vi "Bus Wiring.vi"(6 "Variant in":variant, 7 "Shift Pressed?":bool, 8 "error in (no error)":errorcluster, 10 "QD Combo Box Ref":refnum<vi>, 11 "QD Launch VI Ref":refnum<vi>) -> (0 "error out":errorcluster, 4 "Variant out":variant)   [LabVIEW 2019]
doc: "Attempt to bus wires\n\nDefault Shortcut - [e]"
panel:
  in  "Undo Name":string="Reset to Origin"
  # "Do not change the connector pane of this VI.\n\nSee the block diagram for directions on how to use this template."
  # "Specify the name of the Undo transaction"
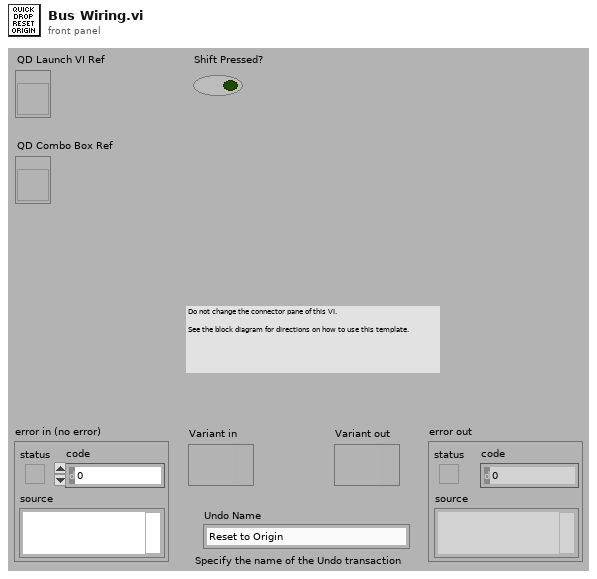
[diagram p1: front panel]
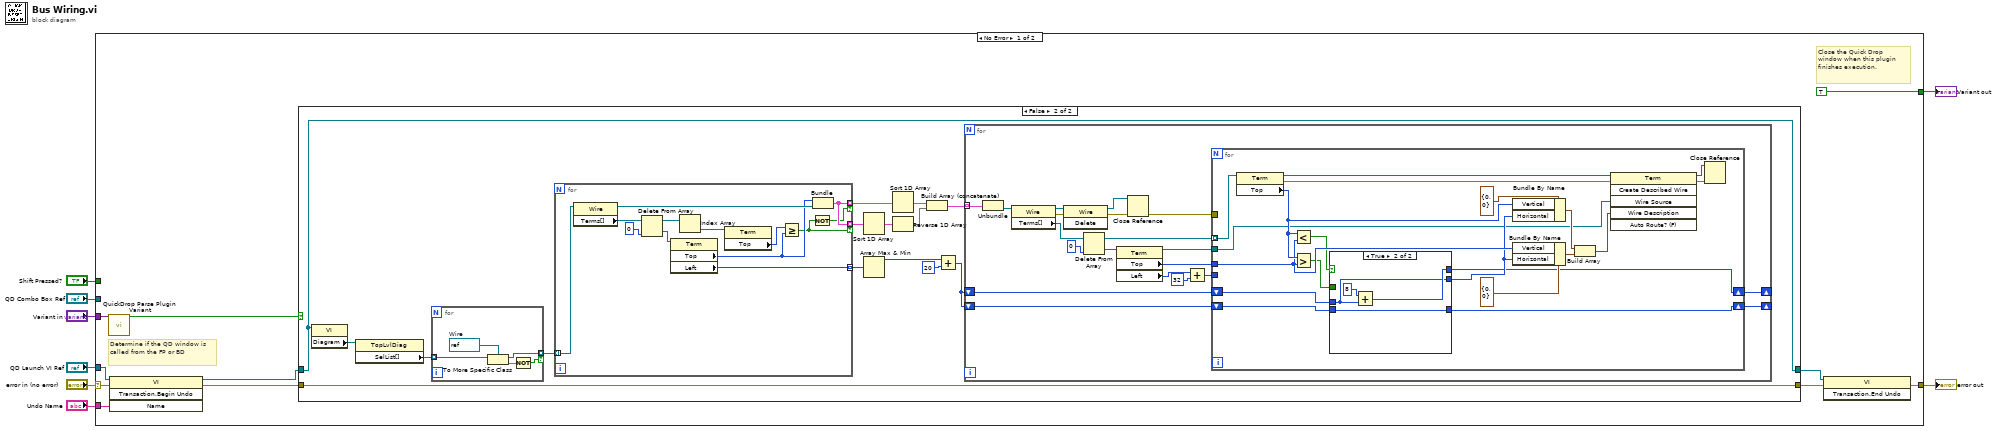
[diagram p0: block diagram]
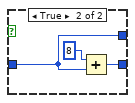
[diagram p4: hidden frame]
diagram:
  n1 = case shown="No Error" "error in (no error)" {
    selector: "error in (no error)" -> [w18 w108]
    tunnel: [w12 w108] -> w7
    tunnel: "QD Launch VI Ref" -> [w17 _]
    tunnel: "Shift Pressed?" -> [_ _]
    tunnel: "QD Combo Box Ref" -> [_ _]
    tunnel: "Variant in" -> [w19 _]
    tunnel: "Undo Name" -> [w16 _]
    tunnel: [TRUE _] -> w1
    frame No Error {
      # "Close the Quick Drop window when this plugin finishes execution."
      # "Determine if the QD window is called from the FP or BD"
      n2 = call <vilib>:"QuickDrop Parse Plugin Variant.vi"("QDKS Variant in"=w19) -> ("QD Launch VI Panel?"=w14:bool)  [unwired: 12 in, 2 out]
      n3 = invoke class="VI" method="Transaction.Begin Undo"(reference=w17, error in=w18, "Name"=w16) -> (reference out=w11:refnum<vi>, error out=w13:errorcluster)  [unwired: 1 in, 2 out]
      n4 = case shown="False" w14 {
        tunnel: w13 -> [w21 w36]
        tunnel: w11 -> [w20 w34]
        tunnel: [w21 w36] -> w10
        tunnel: [w20 w34] -> w9
        frame True {
          # "Do nothing on the front panel."
        }
        frame False {
          n5 = property class="VI"(reference=w34) -> ("Diagram"=w35:refnum<vi>)  [unwired: 1 in, 2 out]
          n6 = property class="TopLvlDiag"(reference=w35) -> ("SelList[]"=w33:refnum<vi>[])  [unwired: 1 in, 2 out]
          n7 = for {
            tunnel: w33 -> [w103] mode=indexing
            tunnel: [w106] -> w32 mode=indexing if=w104
            w107 = refnum<vi> refnum  # Wire
            n8 = To More Specific Class(target class=w107, reference=w103) -> (specific class reference=w106:refnum<vi>, error out=w105:errorcluster)  [unwired: 1 in]
            n9 = Not(x=w105) -> (.not. x?=w104:bool)
          }
          n10 = for {
            tunnel: w32 -> [w49] mode=indexing
            tunnel: [w39] -> w31 mode=indexing if=w38
            tunnel: [w44] -> w28 mode=indexing
            tunnel: [w39] -> w25 mode=indexing if=w37
            n11 = property class="Wire"(reference=w49) -> (reference out=w45:refnum<vi>, "Terms[]"=w46:refnum<vi>[])  [unwired: 1 in, 1 out]
            n12 = Delete From Array(array=w46, index=0) -> (deleted portion=w48:refnum<vi>, array with subset deleted=w43:refnum<vi>[])  [unwired: 1 in]
            n13 = property class="Term"(reference=w48) -> ("Top"=w40:i32, "Left"=w44:i32)  [unwired: 1 in, 2 out]
            n14 = Index Array(array=w43) -> (element=w42:refnum<vi>)  [unwired: 1 in]
            n15 = property class="Term"(reference=w42) -> ("Top"=w41:i32)  [unwired: 1 in, 2 out]
            n16 = Greater Or Equal?(x=w41, y=w40) -> (x >= y?=w37:bool)
            n17 = Not(x=w37) -> (.not. x?=w38:bool)
            n18 = Bundle("Top"=w40, w45) -> (w39:cluster{"Top":i32, refnum<vi>})  [unwired: 1 in]
          }
          n19 = Sort 1D Array(array=w25) -> (sorted array=w24:cluster{"Top":i32, refnum<vi>}[])
          n20 = Array Max & Min(array=w28) -> (max value=w26:i32)  [unwired: 3 out]
          n21 = Sort 1D Array(array=w31) -> (sorted array=w30:cluster{"Top":i32, refnum<vi>}[])
          n22 = Reverse 1D Array(array=w24) -> (reversed array=w22:cluster{"Top":i32, refnum<vi>}[])
          n23 = Build Array (concatenate)(w30, w22) -> (w23:cluster{"Top":i32, refnum<vi>}[])
          n24 = Add(x=w26, y=20 ("x")) -> (x+y=w27:i32)
          n25 = for {
            tunnel: w23 -> [w63] mode=indexing
            shift-right: [w55] -> _
            shift-left: w27 -> [w56]
            shift-right: [w53] -> _
            shift-left: w27 -> [w54]
            n26 = Unbundle(w63) -> (w62:refnum<vi>)  [unwired: 1 out]
            n27 = property class="Wire"(reference=w62) -> (reference out=w60:refnum<vi>, error out=w61:errorcluster, "Terms[]"=w68:refnum<vi>[])  [unwired: 1 in]
            n28 = invoke class="Wire" method="Delete"(reference=w60, error in=w61) -> (reference out=w50:refnum<vi>, error out=w59:errorcluster)  [unwired: 1 in, 1 out]
            n29 = Delete From Array(array=w68, index=0) -> (deleted portion=w67:refnum<vi>, array with subset deleted=w66:refnum<vi>[])  [unwired: 1 in]
            n30 = property class="Term"(reference=w67) -> (reference out=w52:refnum<vi>, "Top"=w58:i32, "Left"=w64:i32)  [unwired: 1 in, 1 out]
            n31 = Close Reference(reference=w50, error in (no error)=w59) -> (error out=w51:errorcluster)
            n32 = Add(x=w64, y=32 ("x")) -> (x+y=w57:i32)
            n33 = for {
              tunnel: w66 -> [w89] mode=indexing
              tunnel: w51 -> [_]
              tunnel: w58 -> [w80]
              tunnel: w57 -> [_]
              shift-right: [w76] -> w55
              shift-left: w56 -> [w75]
              shift-right: [w73] -> w53
              shift-left: w54 -> [w74]
              tunnel: w52 -> [w72]
              n34 = property class="Term"(reference=w89) -> (reference out=w71:refnum<vi>, error out=w70:errorcluster, "Top"=w81:i32)  [unwired: 1 in]
              n35 = Less?(x=w81, y=w80) -> (x < y?=w79:bool)
              n36 = Greater?(x=w81, y=w80) -> (0:w78:bool)
              n37 = case shown="True" w79 {
                tunnel: w78 -> [w94 _]
                tunnel: [w92 w100] -> w77
                tunnel: w75 -> [w90 w100]
                tunnel: [w90 w101] -> w76
                tunnel: w74 -> [w93 w99]
                tunnel: [w91 w99] -> w73
                frame False {
                  n38 = case shown="False" w94 {
                    tunnel: w93 -> [w95 w97]
                    tunnel: [w95 w97] -> w92
                    tunnel: [w95 w96] -> w91
                    frame False {
                    }
                    frame True {
                      n39 = Add(x=8, y=w97) -> (x+y=w96:i32)
                    }
                  }
                }
                frame True {
                  n40 = Add(x=8, y=w100) -> (x+y=w101:i32)
                }
              }
              n41 = Bundle By Name(cluster=cluster{"Vertical":i16, "Horizontal":i16} {"Vertical"=0, "Horizontal"=0}, "Vertical"=w81, "Horizontal"=w77) -> (w87:cluster{"Vertical":i16, "Horizontal":i16})
              n42 = Bundle By Name(cluster=cluster{"Vertical":i16, "Horizontal":i16} {"Vertical"=0, "Horizontal"=0}, "Vertical"=w80, "Horizontal"=w77) -> (w82:cluster{"Vertical":i16, "Horizontal":i16})
              n43 = Build Array(w87, w82) -> (w84:cluster{"Vertical":i16, "Horizontal":i16}[])
              n44 = invoke class="Term" method="Create Described Wire"(reference=w71, error in=w70, "Wire Source"=w72, "Wire Description"=w84) -> (reference out=w86:refnum<vi>, error out=w85:errorcluster)  [unwired: 2 in, 4 out]
              n45 = Close Reference(reference=w86, error in (no error)=w85) -> ()  [unwired: 1 out]
            }
          }
        }
      }
      n46 = invoke class="VI" method="Transaction.End Undo"(reference=w9, error in=w10) -> (error out=w12:errorcluster)  [unwired: 1 in, 2 out]
    }
    frame Error {
    }
  }
  "error out" <- w7
  "Variant out" <- w1
